vi "VariantToProperties.vi"(0 "ChromaAcLoad":refnum<class "ChromaAcLoad.lvclass">, 11 "error in (no error)":errorcluster) -> (4 "ChromaAcLoad":refnum<class "ChromaAcLoad.lvclass">, 6 "Device Properties":T5 {"Phases"."Phase Select" items=["Phase ALL", "Phase A", "Phase B", "Phase C"]}, 8 "Meas":T3, 10 "Configuration Mode":T1(ring), 13 "Measurement Refresh Time (ms)":u32, 14 "Phases":T2(array[cluster]), 15 "error out":errorcluster)   [LabVIEW 2018, in "AcPwrPlugins.lvlib" / "ChromaAcLoad.lvclass"]
doc: "This VI extracts the variant input and converts it into the plugin configuration datatype."
uses:
  ChromaAcLoad.lvclass
  TypeDefs/Device(s)Settings.ctl
  C:/Users/Public/Projects/ICDAS/NistPluggableModules/AcPwr/AcPwrPlugins/AcPwrBaseClass/AcPwrBase.lvclass
  TypeDefs/Measurements.ctl
  TypeDefs/MeasurementType.ctl
  AcPwrBaseClass/AcPwrBase.lvclass/AcPwrBase.ctl
  AcPwrBaseClass/Accessors/Read BaseConfig.vi
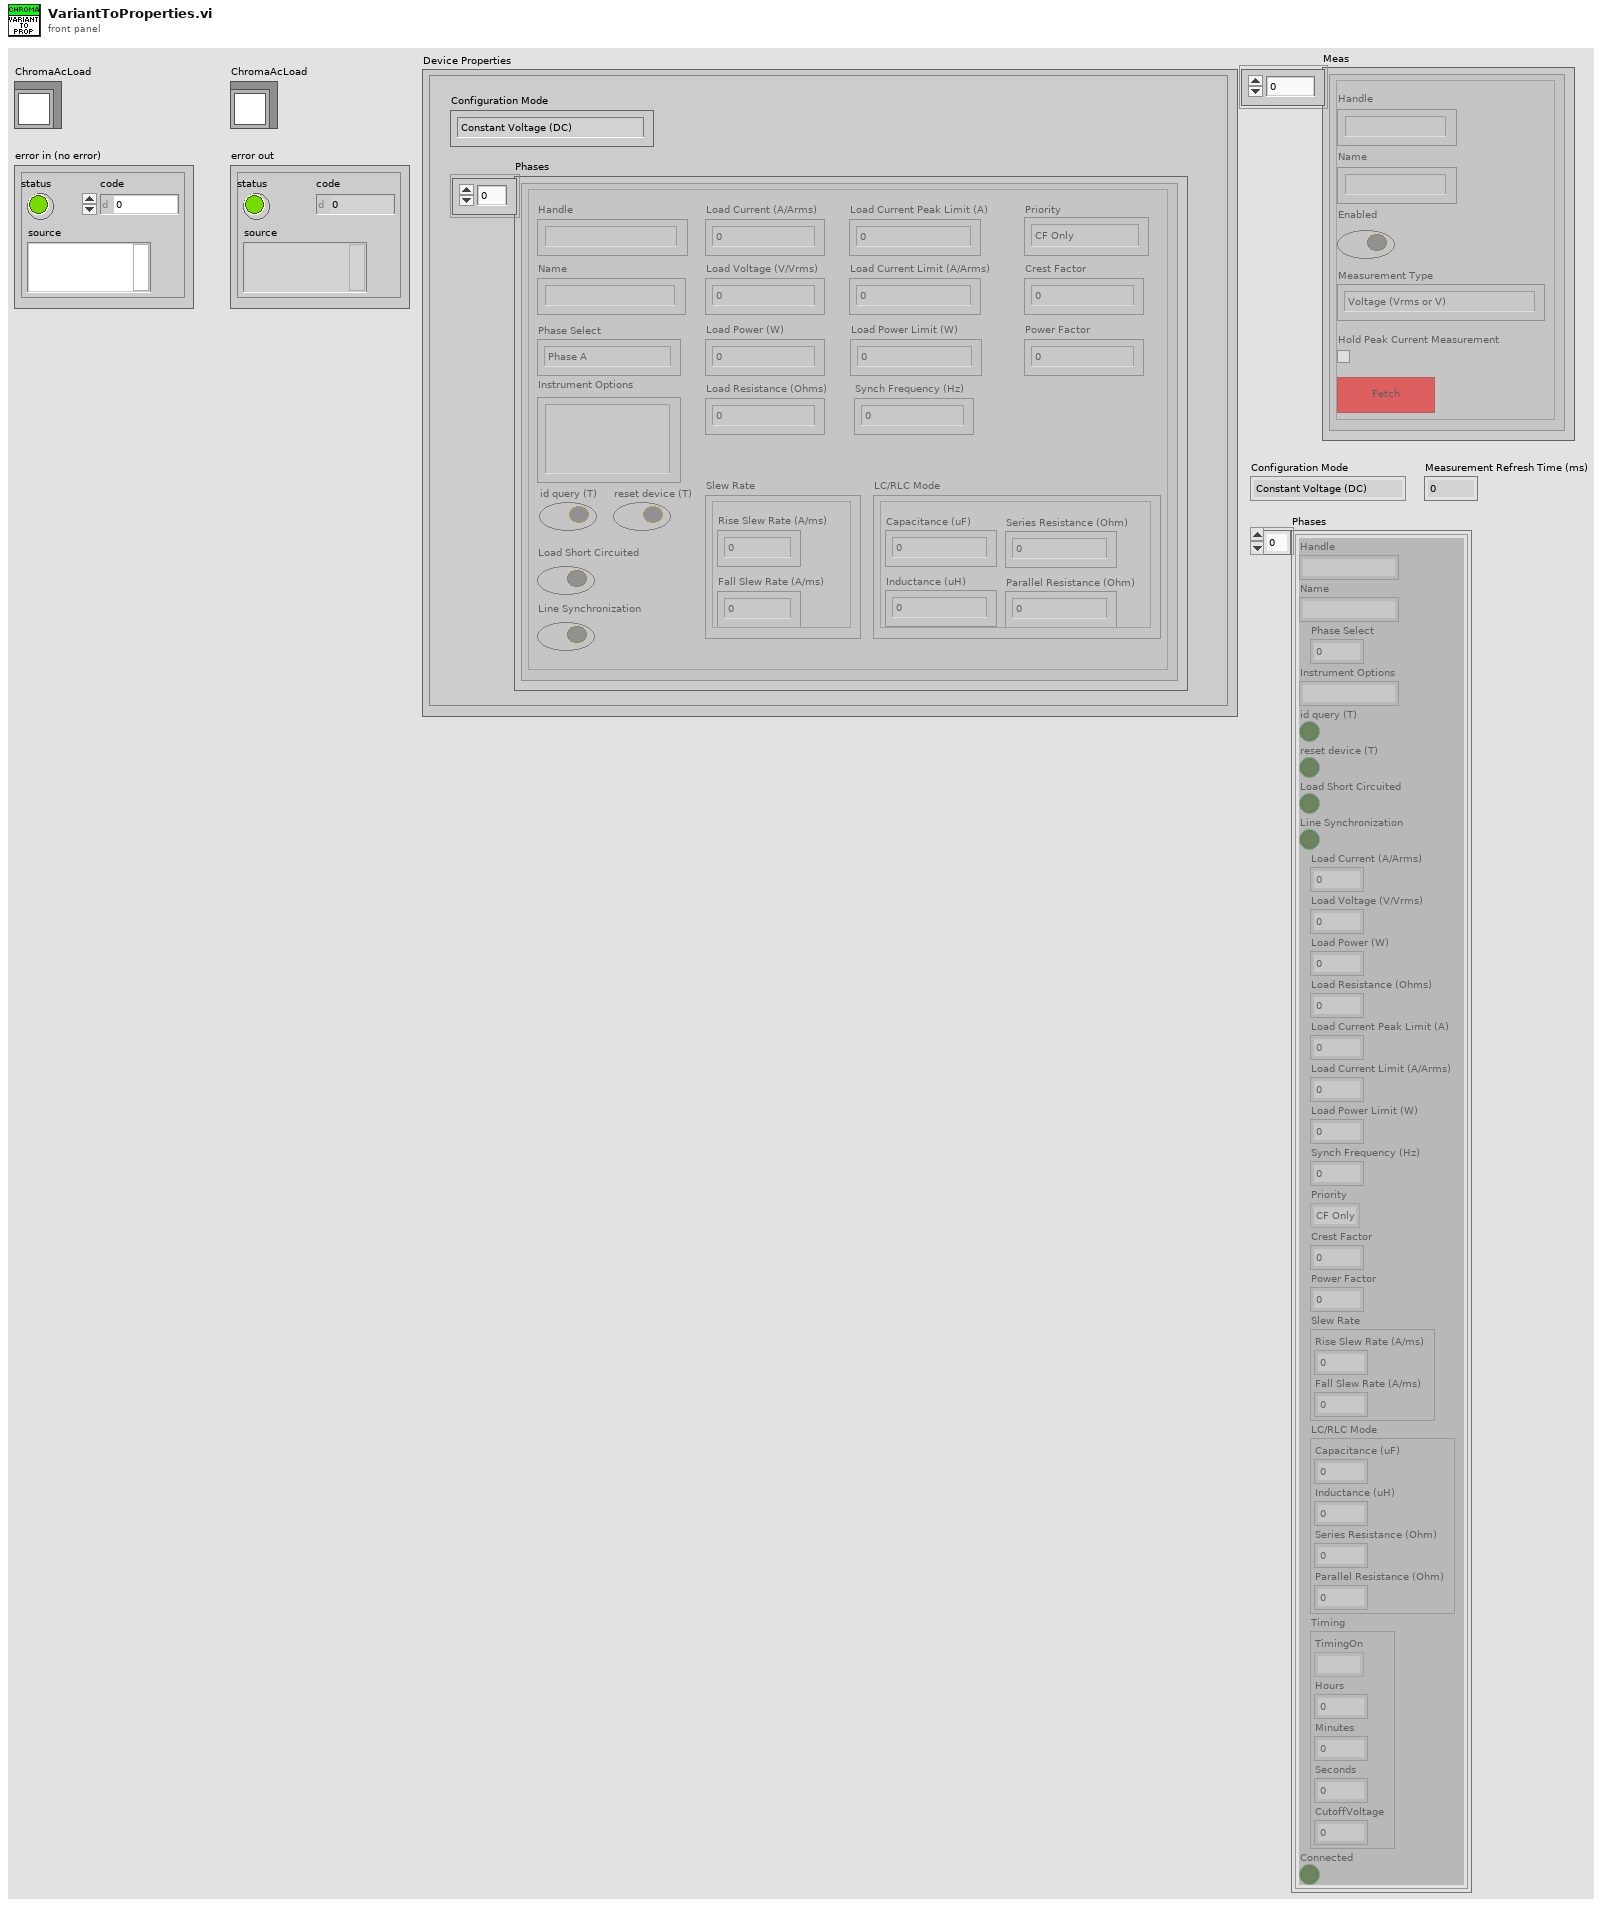
[diagram p1: front panel]
types:
  T1 = enum16{"Constant Voltage (DC)", "Constant Power (DC)", "Constant Power (AC)", "Constant Current (DC)", "Constant Current (AC)", "Constant Resistance (DC)", "Constant Resistance (AC)", "Rectified Mode (DC)", "Inrush (AC)", "RLC CP (AC)", "RLC (AC)"}
  T2 = cluster{"Handle":string, "Name":string, "Phase Select":i32, "Instrument Options":string, "id query (T)":bool, "reset device (T)":bool, "Load Short Circuited":bool, "Line Synchronization":bool, "Load Current (A/Arms)":dbl, "Load Voltage (V/Vrms)":dbl, "Load Power (W)":dbl, "Load Resistance (Ohms)":dbl, "Load Current Peak Limit (A)":dbl, "Load Current Limit (A/Arms)":dbl, "Load Power Limit (W)":dbl, "Synch Frequency (Hz)":dbl, "Priority":enum16{"CF Only", "PF Only", "Both (CF)", "Both (PF)"}, "Crest Factor":dbl, "Power Factor":dbl, "Slew Rate":cluster{"Rise Slew Rate (A/ms)":i32, "Fall Slew Rate (A/ms)":i32}, "LC/RLC Mode":cluster{"Capacitance (uF)":i32, "Inductance (uH)":i32, "Series Resistance (Ohm)":dbl, "Parallel Resistance (Ohm)":dbl}, "Timing":cluster{"TimingOn":enum16{""}, "Hours":u32, "Minutes":u32, "Seconds":dbl, "CutoffVoltage":dbl}, "Connected":bool}[]
  T3 = typedef "AcPwrPlugins.lvlib/ChromaAcLoad.lvclass/Measurements.ctl" = cluster{"Handle":string, "Name":string, "Enabled":bool, "Measurement Value":dbl, "Hold Peak Current Measurement":bool, "btnMeasFetch":bool, "ProtectionStatusString":string, "Measurement Type":T4}[]
  T4 = typedef "AcPwrPlugins.lvlib/ChromaAcLoad.lvclass/MeasurementType.ctl" = enum16{"Voltage (Vrms or V)", "Current (Arms or A)", "Power (W)", "Peak Voltage (V)", "Peak Current (A)", "Peak Power (W)", "Frequency (Hz)", "Resistance (Ohms)", "Voltage Overshoot (V)", "Positive Peak Current (A)", "Voltage Undershoot (V)", "Negative Peak Current (A)", "Apparent Power (VA)", "Reacitive Power (VAR)", "Voltage THD", "Power Factor", "Current's Crest Factor"}
  T5 = typedef "AcPwrPlugins.lvlib/ChromaAcLoad.lvclass/Device(s)Settings.ctl" = cluster{"Configuration Mode":enum16{"Constant Voltage (DC)", "Constant Power (DC)", "Constant Power (AC)", "Constant Current (DC)", "Constant Current (AC)", "Constant Resistance (DC)", "Constant Resistance (AC)", "Rectified Mode (DC)", "Inrush (AC)", "RLC CP (AC)", "RLC (AC)"}, "Phases":cluster{"Handle":string, "Name":string, "Phase Select":i32, "Instrument Options":string, "id query (T)":bool, "reset device (T)":bool, "Load Short Circuited":bool, "Line Synchronization":bool, "Load Current (A/Arms)":dbl, "Load Voltage (V/Vrms)":dbl, "Load Power (W)":dbl, "Load Resistance (Ohms)":dbl, "Load Current Peak Limit (A)":dbl, "Load Current Limit (A/Arms)":dbl, "Load Power Limit (W)":dbl, "Synch Frequency (Hz)":dbl, "Priority":enum16{"CF Only", "PF Only", "Both (CF)", "Both (PF)"}, "Crest Factor":dbl, "Power Factor":dbl, "Slew Rate":cluster{"Rise Slew Rate (A/ms)":i32, "Fall Slew Rate (A/ms)":i32}, "LC/RLC Mode":cluster{"Capacitance (uF)":i32, "Inductance (uH)":i32, "Series Resistance (Ohm)":dbl, "Parallel Resistance (Ohm)":dbl}, "Timing":cluster{"TimingOn":enum16{""}, "Hours":u32, "Minutes":u32, "Seconds":dbl, "CutoffVoltage":dbl}, "Connected":bool}[], "MeasName":string}
  T6 = typedef "AcPwrPlugins.lvlib/AcPwrBase.lvclass/BaseConfig.ctl" = cluster{"Frequency":dbl, "FrequencyRange":dbl[], "Phases":T7[], "Name":string, "PluginConfigVariant":variant, "PluginMeasVariant":variant}
  T7 = typedef "AcPwrPlugins.lvlib/AcPwrBase.lvclass/Phase.ctl" = cluster{"Name":string, "Enabled":bool, "VoltageLevel":dbl, "Handle":string, "VoltageRange":dbl[], "Connected":bool, "CurrentLimit":dbl, "Waveform":string}
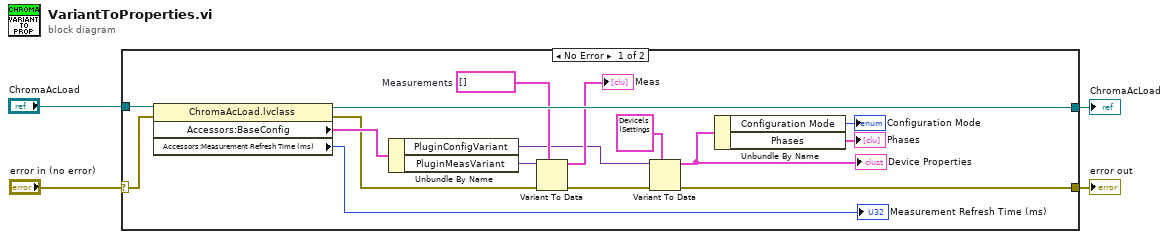
[diagram p0: block diagram]
diagram:
  n1 = case shown="No Error" "error in (no error)" {
    selector: "error in (no error)" -> [w17 w22]
    tunnel: [w20 w22] -> w3
    tunnel: "ChromaAcLoad" -> [w18 w21]
    tunnel: [w16 w21] -> w1
    frame No Error {
      w11 = T3 []  # Measurements
      n2 = property class="ChromaAcLoad.lvclass"(reference=w18, error in=w17) -> (reference out=w16:refnum<class "ChromaAcLoad.lvclass">, error out=w14:errorcluster, "Accessors:BaseConfig"=w15:T6, "Accessors:Measurement Refresh Time (ms)"=→"Measurement Refresh Time (ms)":u32)
      n3 = Unbundle By Name(w15) -> ("PluginConfigVariant"=w9:variant, "PluginMeasVariant"=w13:variant)
      n4 = Variant To Data(error in=w14, type=w11, Variant=w13) -> (data=→"Meas":T3, error out=w12:errorcluster)
      n5 = Variant To Data(error in=w12, type=T5 {"Configuration Mode"=enum."Constant Voltage (DC)", "Phases"=[], "MeasName"=""} ("Chroma"), Variant=w9) -> (data=w8:T5, error out=w20:errorcluster)
      "Device Properties" <- w8
      n6 = Unbundle By Name(w8) -> ("Configuration Mode"=→"Configuration Mode":T1, "Phases"=→"Phases":T2)
    }
    frame Error {
    }
  }
  "error out" <- w3
  "ChromaAcLoad" <- w1
